vi "convert data to decibels start.vi"(7 "data in":dbl[](array[numeric]), 11 "Lin/dB":bool) -> (8 "data out":dbl[](array[numeric]))   [LabVIEW 2019]
doc: "this subvi either lets data pass through unaffected, or converts it to Decibels by taking 10*log(data). We do this for plotting so that we can see the noise. Note this is power data so we use 10 in the dB formula, not 20 like for voltages directly."
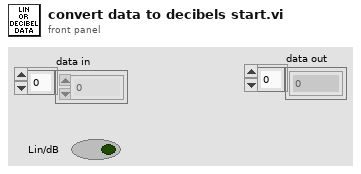
[diagram p1: front panel]
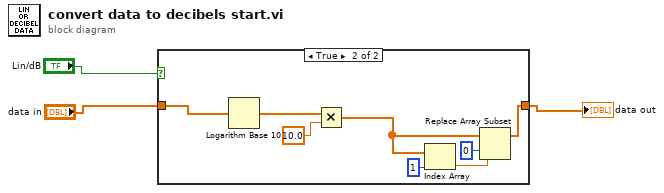
[diagram p0: block diagram]
diagram:
  n1 = case shown="True" "Lin/dB" {
    tunnel: "data in" -> [w4 w9]
    tunnel: [w4 w5] -> w2
    frame False {
    }
    frame True {
      n2 = Logarithm Base 10(1:w9) -> (0:w7:dbl[])
      n3 = Multiply(x=w7, y=10.0) -> (x*y=w6:dbl[])
      n4 = Index Array(array=w6, index=1) -> (element=w12:dbl)
      n5 = Replace Array Subset(array=w6, new element=w12, index=0) -> (w5:dbl[])
    }
  }
  "data out" <- w2
